vi "AddBus.vi"(7 "ShowPanels?":bool, 8 "ErrorArray In":errorcluster[](array[cluster]), 11 "BusClass In":refnum<class "Bus.lvclass">) -> (0 "ErrorArray Out":errorcluster[](array[cluster]), 2 "UserEvents":T5, 3 "BusClass Out":refnum<class "Bus.lvclass">)   [LabVIEW 2017, in "Bus_class.lvlib" / "Bus.lvclass"]
uses:
  Bus.lvclass
  Modules/EventModule/Protected/Broadcasts/clBroadcastEvents.ctl
  Modules/EventModule/Protected/clEventType.ctl
  Modules/PmuImpairModule/Protected/Broadcasts/clBroadcastEvents.ctl
  Modules/PmuImpairModule/Protected/clEventType.ctl
  Modules/NetworkImpairmentModule/Protected/Broadcasts/clBroadcastEvents.ctl
  Modules/NetworkImpairmentModule/Protected/clEventType.ctl
  Modules/FlagImpairModule/Protected/Broadcasts/clBroadcastEvents.ctl
  Modules/FlagImpairModule/Protected/clEventType.ctl
  <userlib>/NIST/ModuleAdminLib/ModuleAdmin/ModuleAdmin.lvclass
  Modules/EventModule/EventModule.lvlib
  Modules/PmuImpairModule/PmuImpairModule.lvlib
  <userlib>/NIST/NISTErrorLib/NISTErrorLib.lvlib
  Modules/NetworkImpairmentModule/NetworkImpairmentModule.lvlib
  Modules/FlagImpairModule/FlagImpairModule.lvlib
  Bus_class.lvlib
panel:
  # "If you want to add other Broadcast Events, open this typedef, copy an existing event and rename it to your event name.\n\nNext create a typedef for the  data and put it into PublicAPI/Arguments/Broadcasts"
  # "If you want to add other Broadcast Events, open this typedef, copy an existing event and rename it to your event name.\n\nNext create an \"arg\" typedef for the  data and put it into PublicAPI/Arguments/Broadcasts\n\nAfter that, you will need to create a new roadcast vi in Protected/Broadcast.  Look at DidInit.vi or the reportError.vi as examples."
  # "If you want to add other Broadcast Events, open this typedef, copy an existing event and rename it to your event name.\n\nNext create an \"arg\" typedef for the  data and put it into PublicAPI/Arguments/Broadcasts\n\nAfter that, you will need to create a new roadcast vi in Protected/Broadcast.  Look at DidInit.vi or the reportError.vi as examples."
  # "If you want to add other Broadcast Events, open this typedef, copy an existing event and rename it to your event name.\n\nNext create an \"arg\" typedef for the  data and put it into PublicAPI/Arguments/Broadcasts\n\nAfter that, you will need to create a new roadcast vi in Protected/Broadcast.  Look at DidInit.vi or the reportError.vi as examples."
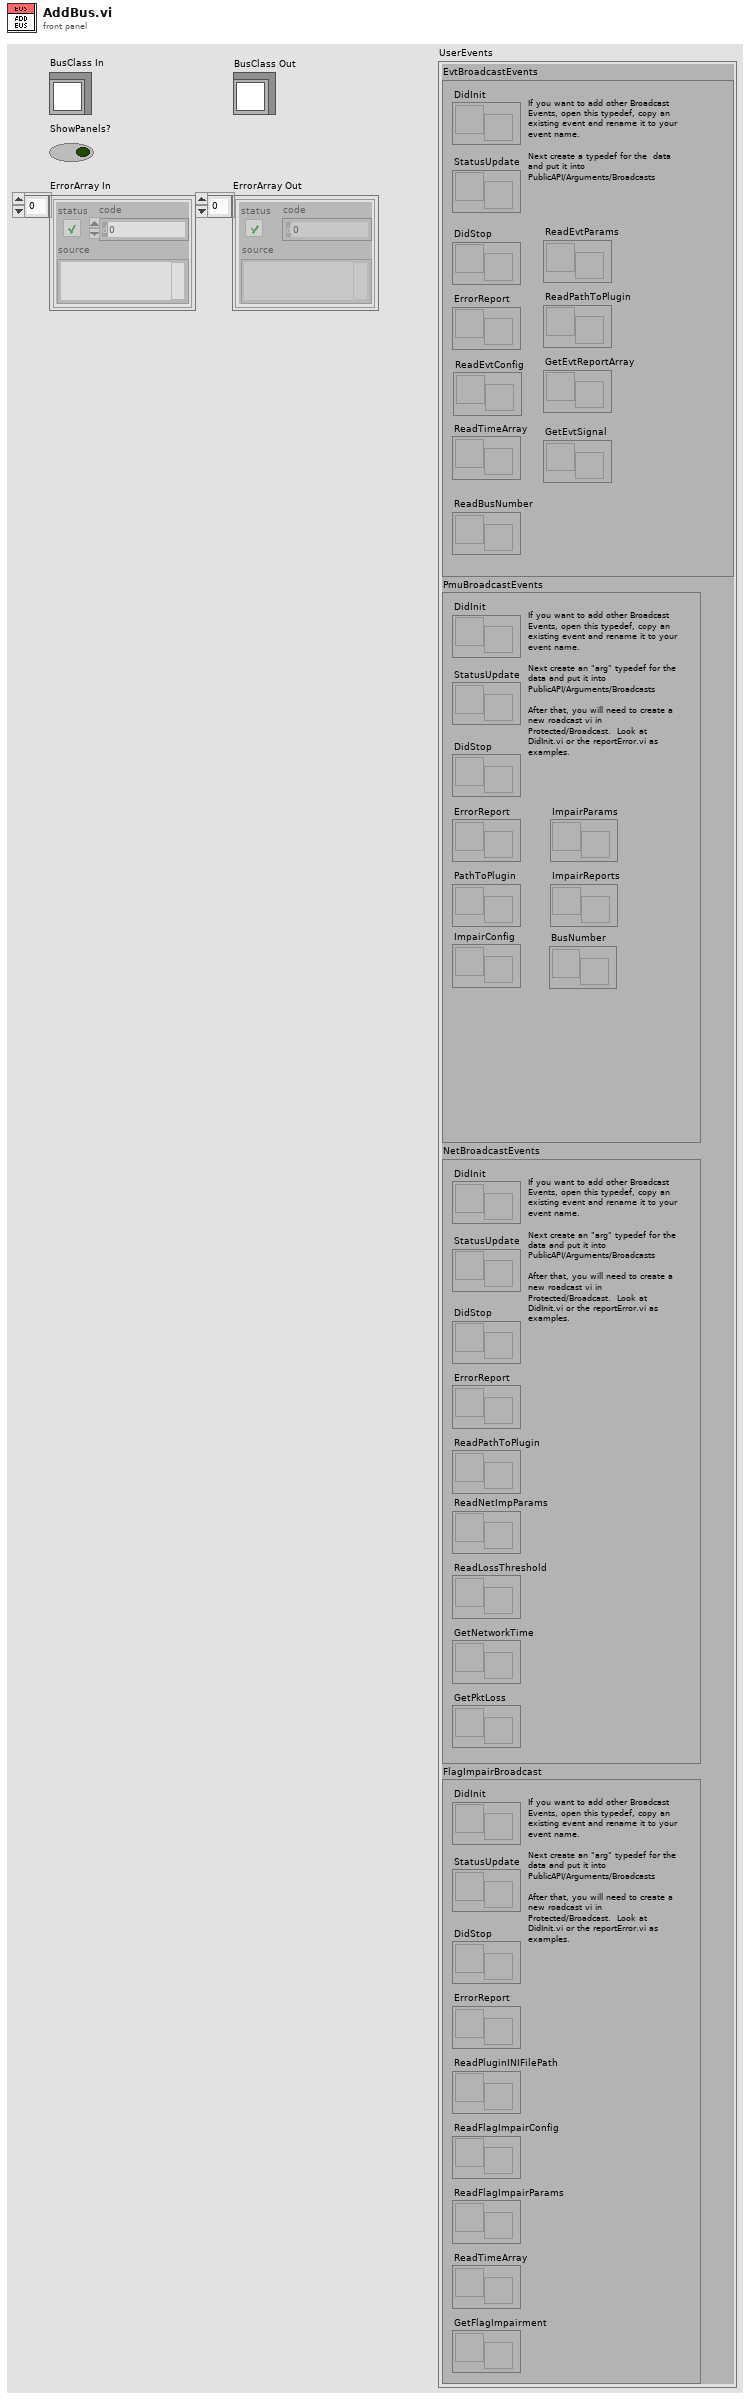
[diagram p1: front panel]
types:
  T1 = typedef "EventModule.lvlib/clBroadcastEvents.ctl" = cluster{"DidInit":refnum<user-event>, "StatusUpdate":refnum<user-event>, "ErrorReport":refnum<user-event>, "DidStop":refnum<user-event>, "ReadEvtConfig":refnum<user-event>, "ReadTimeArray":refnum<user-event>, "ReadEvtParams":refnum<user-event>, "GetEvtReportArray":refnum<user-event>, "ReadPathToPlugin":refnum<user-event>, "GetEvtSignal":refnum<user-event>, "ReadBusNumber":refnum<user-event>}
  T2 = typedef "PmuImpairModule.lvlib/clBroadcastEvents.ctl" = cluster{"DidInit":refnum<user-event>, "StatusUpdate":refnum<user-event>, "ErrorReport":refnum<user-event>, "DidStop":refnum<user-event>, "ImpairConfig":refnum<user-event>, "ImpairParams":refnum<user-event>, "ImpairReports":refnum<user-event>, "PathToPlugin":refnum<user-event>, "BusNumber":refnum<user-event>}
  T3 = typedef "NetworkImpairmentModule.lvlib/clBroadcastEvents.ctl" = cluster{"DidInit":refnum<user-event>, "StatusUpdate":refnum<user-event>, "ErrorReport":refnum<user-event>, "DidStop":refnum<user-event>, "ReadNetImpParams":refnum<user-event>, "ReadLossThreshold":refnum<user-event>, "GetNetworkTime":refnum<user-event>, "GetPktLoss":refnum<user-event>, "ReadPathToPlugin":refnum<user-event>}
  T4 = typedef "FlagImpairModule.lvlib/clBroadcastEvents.ctl" = cluster{"DidInit":refnum<user-event>, "StatusUpdate":refnum<user-event>, "ErrorReport":refnum<user-event>, "DidStop":refnum<user-event>, "ReadFlagImpairConfig":refnum<user-event>, "ReadPluginINIFilePath":refnum<user-event>, "ReadFlagImpairParams":refnum<user-event>, "ReadTimeArray":refnum<user-event>, "GetFlagImpairment":refnum<user-event>}
  T5 = cluster{"EvtBroadcastEvents":T1, "PmuBroadcastEvents":T2, "NetBroadcastEvents":T3, "FlagImpairBroadcast":T4}
  T6 = cluster{"clBroadcastEvents":T1, "clBroadcastEvents":T2, "clBroadcastEvents":T3, "FlagImpairBroadcast":T4}
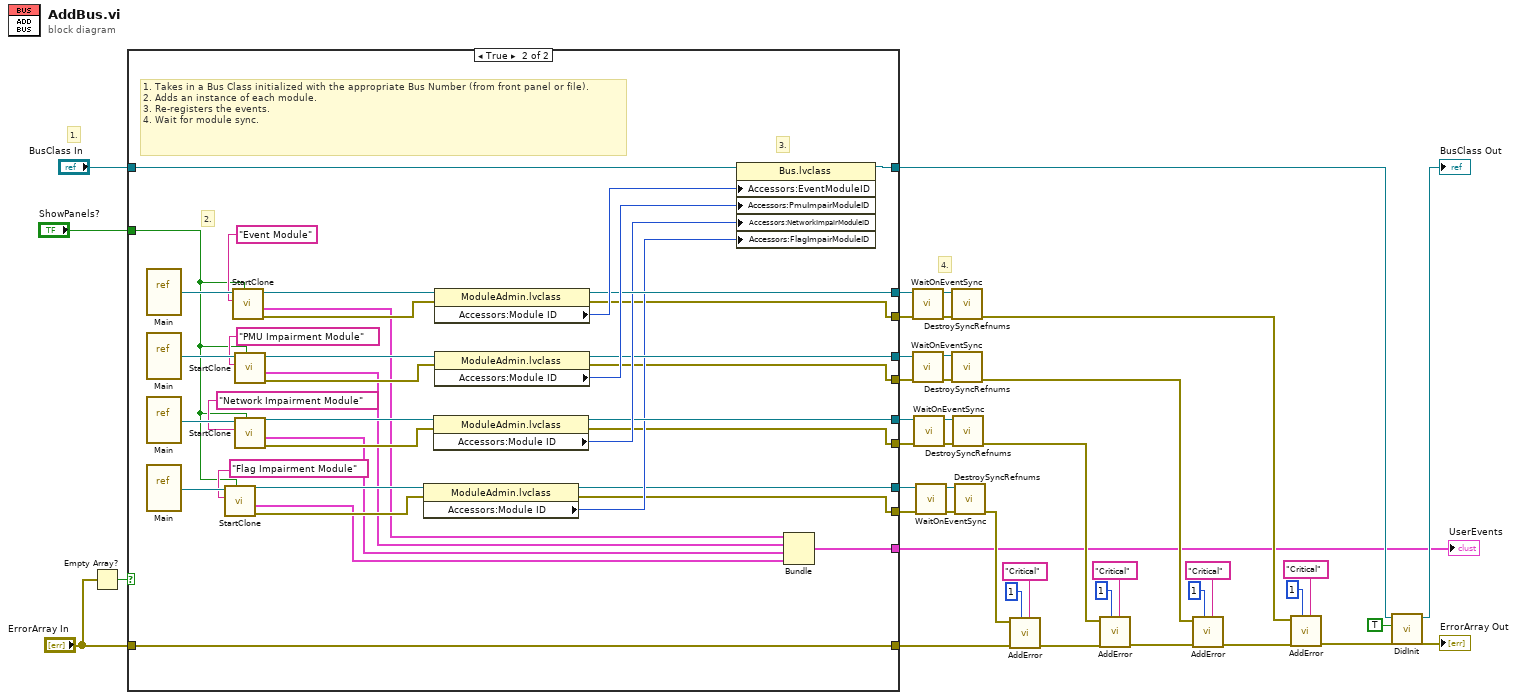
[diagram p0: block diagram]
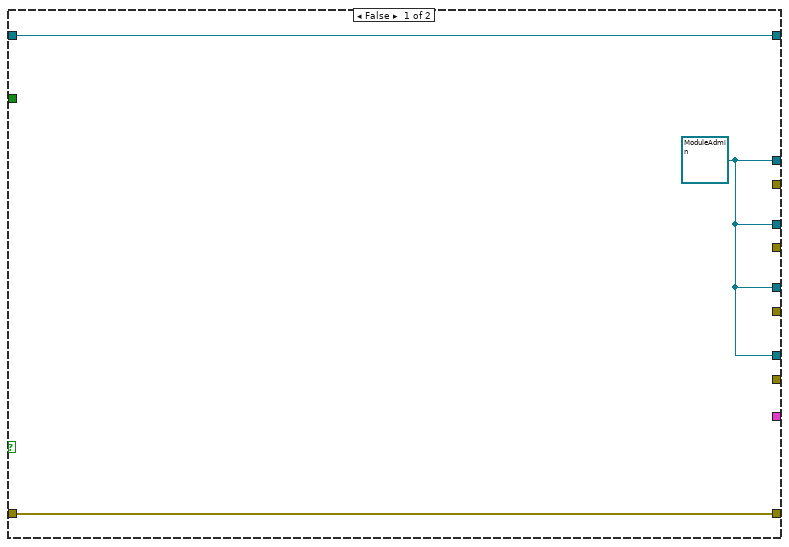
[diagram p2: hidden frame]
diagram:
  # "4."
  # "1."
  n1 = Empty Array?(array="ErrorArray In") -> (empty?=w42:bool)
  n2 = case shown="True" w42 {
    tunnel: [w44 w49] -> w2
    tunnel: "BusClass In" -> [w45 w80]
    tunnel: [w45 w76] -> w5
    tunnel: "ErrorArray In" -> [w44 w49]
    tunnel: [w43 w70] -> w37
    tunnel: [w43 w64] -> w32
    tunnel: [w43 w63] -> w31
    tunnel: [w43 w57] -> w28
    tunnel: [_ w56] -> w27
    tunnel: [_ w55] -> w26
    tunnel: [_ w54] -> w25
    tunnel: [_ w53] -> w24
    tunnel: [_ w47] -> w3
    tunnel: "ShowPanels?" -> [_ w46]
    frame False {
      w43 = refnum<class "ModuleAdmin.lvclass"> refnum ("ModuleAdmin")
    }
    frame True {
      # "3."
      # "2."
      # "1. Takes in a Bus Class initialized with the appropriate Bus Number (from front panel or file).\n2. Adds an instance of each module.\n3. Re-registers the events.\n4. Wait for module sync."
      n3 = vi-ref "Main.vi"() -> (w82:refnum<vi>)
      n4 = vi-ref "Main.vi"() -> (w73:refnum<vi>)
      n5 = vi-ref "Main.vi"() -> (w67:refnum<vi>)
      n6 = vi-ref "Main.vi"() -> (w62:refnum<vi>)
      n7 = call "StartClone.vi"("ShowPanel?"=w46, "ModuleName"="Flag Impairment Module", "VI Refnum"=w62) -> ("error out"=w61:errorcluster, "FlagImpairBroadcast"=w48:T4, "ModuleAdmin"=w60:refnum<class "ModuleAdmin.lvclass">)  [unwired: 6 in]
      n8 = call "StartClone.vi"("ShowPanel? (f)"=w46, "ModuleName"="Event Module", "VI Refnum"=w82) -> ("error out"=w78:errorcluster, "clBroadcastEvents"=w52:T1, "ModuleAdmin"=w77:refnum<class "ModuleAdmin.lvclass">)  [unwired: 6 in]
      n9 = call "StartClone.vi"("ShowPanel? (f)"=w46, "ModuleName"="PMU Impairment Module", "VI Refnum"=w73) -> ("error out"=w71:errorcluster, "clBroadcastEvents"=w50:T2, "ModuleAdmin"=w75:refnum<class "ModuleAdmin.lvclass">)  [unwired: 6 in]
      n10 = call "StartClone.vi"("ShowPanel? (f)"=w46, "ModuleName"="Network Impairment Module", "VI Refnum"=w67) -> ("error out"=w68:errorcluster, "clBroadcastEvents"=w51:T3, "ModuleAdmin"=w69:refnum<class "ModuleAdmin.lvclass">)  [unwired: 6 in]
      n11 = property class="ModuleAdmin.lvclass"(reference=w60, error in=w61) -> (reference out=w57:refnum<class "ModuleAdmin.lvclass">, error out=w53:errorcluster, "Accessors:Module ID"=w58:i32)
      n12 = property class="ModuleAdmin.lvclass"(reference=w69, error in=w68) -> (reference out=w63:refnum<class "ModuleAdmin.lvclass">, error out=w54:errorcluster, "Accessors:Module ID"=w65:i32)
      n13 = property class="ModuleAdmin.lvclass"(reference=w77, error in=w78) -> (reference out=w70:refnum<class "ModuleAdmin.lvclass">, error out=w56:errorcluster, "Accessors:Module ID"=w79:i32)
      n14 = property class="ModuleAdmin.lvclass"(reference=w75, error in=w71) -> (reference out=w64:refnum<class "ModuleAdmin.lvclass">, error out=w55:errorcluster, "Accessors:Module ID"=w74:i32)
      n15 = property class="Bus.lvclass"(reference=w80, "Accessors:EventModuleID"=w79, "Accessors:PmuImpairModuleID"=w74, "Accessors:NetworkImpairModuleID"=w65, "Accessors:FlagImpairModuleID"=w58) -> (reference out=w76:refnum<class "Bus.lvclass">)  [unwired: 1 in, 1 out]
      n16 = Bundle("clBroadcastEvents"=w52, "clBroadcastEvents"=w50, "clBroadcastEvents"=w51, "FlagImpairBroadcast"=w48) -> (w47:T6)  [unwired: 1 in]
    }
  }
  "UserEvents" <- w3
  n17 = call <userlib>:"WaitOnEventSync.vi"("error in (no error)"=w27, "ModuleAdmin"=w37) -> ("error out"=w36:errorcluster, "ModuleAdmin"=w39:refnum<class "ModuleAdmin.lvclass">)  [unwired: 8 in]
  n18 = call <userlib>:"WaitOnEventSync.vi"("error in (no error)"=w26, "ModuleAdmin"=w32) -> ("error out"=w35:errorcluster, "ModuleAdmin"=w38:refnum<class "ModuleAdmin.lvclass">)  [unwired: 8 in]
  n19 = call <userlib>:"WaitOnEventSync.vi"("error in (no error)"=w25, "ModuleAdmin"=w31) -> ("error out"=w34:errorcluster, "ModuleAdmin"=w33:refnum<class "ModuleAdmin.lvclass">)  [unwired: 8 in]
  n20 = call <userlib>:"WaitOnEventSync.vi"("error in (no error)"=w24, "ModuleAdmin"=w28) -> ("error out"=w29:errorcluster, "ModuleAdmin"=w30:refnum<class "ModuleAdmin.lvclass">)  [unwired: 8 in]
  n21 = call <userlib>:"DestroySyncRefnums.vi"("error in (no error)"=w36, "ModuleAdmin"=w39) -> ("error out"=w9:errorcluster)  [unwired: 9 in]
  n22 = call <userlib>:"DestroySyncRefnums.vi"("error in (no error)"=w35, "ModuleAdmin"=w38) -> ("error out"=w11:errorcluster)  [unwired: 9 in]
  n23 = call <userlib>:"DestroySyncRefnums.vi"("error in (no error)"=w34, "ModuleAdmin"=w33) -> ("error out"=w13:errorcluster)  [unwired: 9 in]
  n24 = call <userlib>:"DestroySyncRefnums.vi"("error in (no error)"=w29, "ModuleAdmin"=w30) -> ("error out"=w15:errorcluster)  [unwired: 9 in]
  n25 = call <userlib>:"AddError.vi"("Severity"="Critical" ("String"), "Priority"=u8 1, "ErrorArray"=w2, "error in (no error)"=w15) -> ("ErrorArray"=w14:errorcluster[])  [unwired: 6 in, 1 out]
  n26 = call <userlib>:"AddError.vi"("Severity"="Critical" ("String"), "Priority"=u8 1, "ErrorArray"=w14, "error in (no error)"=w13) -> ("ErrorArray"=w12:errorcluster[])  [unwired: 6 in, 1 out]
  n27 = call <userlib>:"AddError.vi"("Severity"="Critical" ("String"), "Priority"=u8 1, "ErrorArray"=w12, "error in (no error)"=w11) -> ("ErrorArray"=w10:errorcluster[])  [unwired: 6 in, 1 out]
  n28 = call <userlib>:"AddError.vi"("Severity"="Critical" ("String"), "Priority"=u8 1, "ErrorArray"=w10, "error in (no error)"=w9) -> ("ErrorArray"=w8:errorcluster[])  [unwired: 6 in, 1 out]
  n29 = call "DidInit.vi"("ErrorArray"=w8, "Init?"=TRUE, "Bus"=w5) -> ("ErrorArray"=→"ErrorArray Out":errorcluster[], "Bus"=→"BusClass Out":refnum<class "Bus.lvclass">)  [unwired: 7 in]
